vi "Waveform_to_xy.vi"(11 "Magnitude":waveform(dbl)) -> (3 "XY Pairs":cluster{"Array":dbl[], "Y":dbl[]})   [LabVIEW 2015]
uses:
  <vilib>/Waveform/WDTOps.llb/WDT Get Waveform Time Array DBL.vi
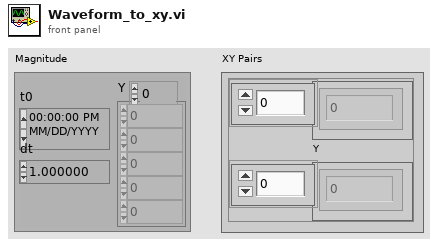
[diagram p1: front panel]
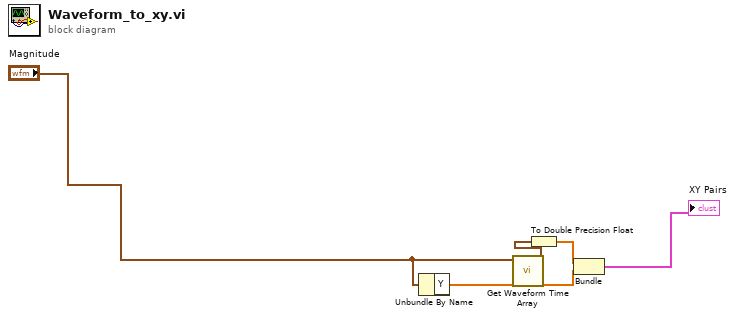
[diagram p0: block diagram]
diagram:
  n1 = Unbundle By Name("Magnitude") -> ("Y"=w4:dbl[])
  n2 = call-poly <vilib>:"Get Waveform Time Array.vi"("waveform in"="Magnitude") -> ("X array"=w1:timestamp[])  [unwired: 9 in, 1 out]
  n3 = To Double Precision Float(number=w1) -> (double precision float=w3:dbl[])
  n4 = Bundle(w3, "Y"=w4) -> (→"XY Pairs":cluster{dbl[], "Y":dbl[]})  [unwired: 1 in]
